vi "tearDown.vi"(8 "error in (no error)":errorcluster, 11 "reference in":refnum<class "Static TestSuite.lvclass">) -> (0 "error out":errorcluster, 3 "reference out":refnum<class "Static TestSuite.lvclass">)   [LabVIEW 2013, in "Static TestSuite.lvclass"]
uses:
  Static TestSuite.lvclass
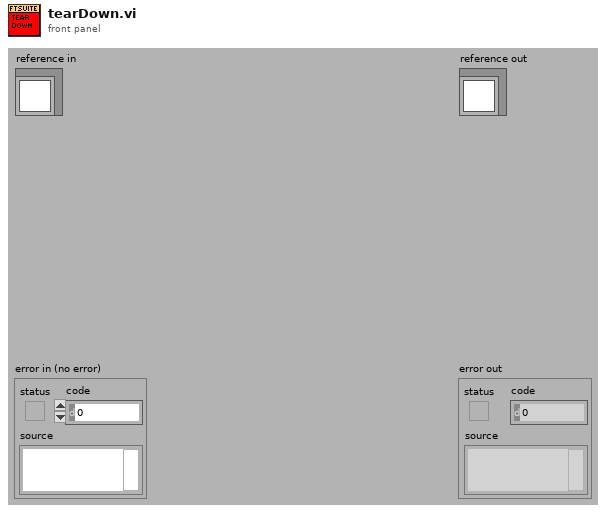
[diagram p1: front panel]
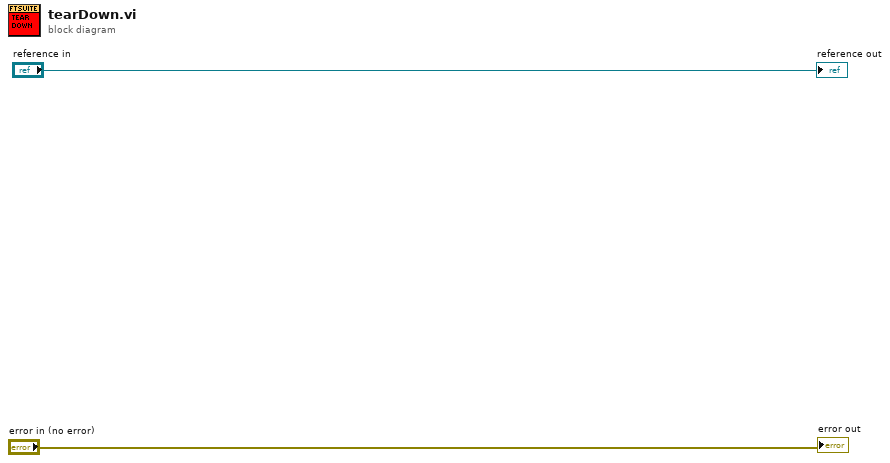
[diagram p0: block diagram]
diagram:
  "error out" <- "error in (no error)"
  "reference out" <- "reference in"
